vi "Random Seed for Parallel Loop.vi"(9 "Iteration":i32, 11 "Seed in (-1)":i32=-1) -> (3 "Seed out":i32)   [LabVIEW 2021, in "Math.lvlib"]
uses:
  Math.lvlib
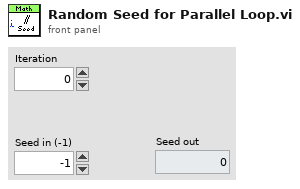
[diagram p1: front panel]
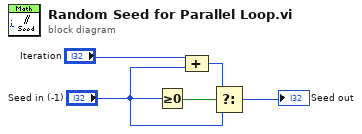
[diagram p0: block diagram]
diagram:
  n1 = Greater Or Equal To 0?(x="Seed in (-1)") -> (x >= 0?=w2:bool)
  n2 = Compound Arithmetic op=ADD("Iteration", "Seed in (-1)") -> (w3:i32)
  n3 = Select(t=w3, s=w2, f="Seed in (-1)") -> (s? t:f=→"Seed out":i32)
